vi "readEnc.vi"(0 "SPI Config In":T2) -> (1 "SPI Config Out":T2, 2 "Data Out":T1)   [LabVIEW 2019]
uses:
  SPI/SPI Config.ctl
panel:
  in  "Data Out Reference":T1
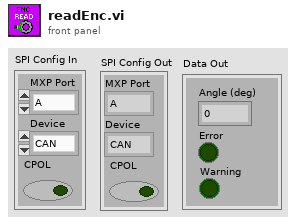
[diagram p1: front panel]
types:
  T1 = cluster{"Angle (deg)":fxp<+,32,16>, "Error":bool, "Warning":bool}
  T2 = typedef "SPI Config.ctl" = cluster{"MXP Port":enum16{"A", "B"}, "Device":enum16{"CAN", "ENC", "IMU1", "IMU2"}, "CPOL":bool}
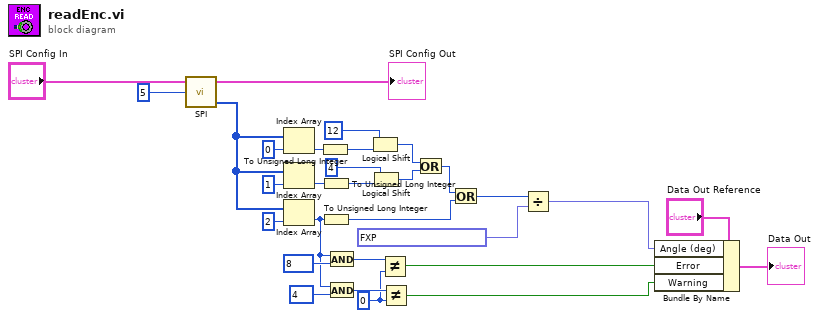
[diagram p0: block diagram]
diagram:
  w6 = u8 0 ("y")
  n1 = call "SPI.vi"("Frames to Write"=u8 5, "SPI Config In"="SPI Config In") -> ("Data Read"=w24:u8[], "SPI Config Out"=→"SPI Config Out":T2)  [unwired: 1 in, 1 out]
  n2 = Index Array(array=w24, index=0) -> (element=w23:u8)
  n3 = Index Array(array=w24, index=1) -> (element=w22:u8)
  n4 = Index Array(array=w24, index=2) -> (element=w10:u8)
  n5 = To Unsigned Long Integer(number=w23) -> (unsigned 32bit integer=w21:u32)
  n6 = To Unsigned Long Integer(number=w22) -> (unsigned 32bit integer=w20:u32)
  n7 = To Unsigned Long Integer(number=w10) -> (unsigned 32bit integer=w14:u32)
  n8 = And(x=w10, y=u8 8) -> (x .and. y?=w8:u8)
  n9 = And(x=w10, y=u8 4) -> (x .and. y?=w7:u8)
  n10 = Logical Shift(y=i16 12, x=w21) -> (x << y=w17:u32)
  n11 = Logical Shift(y=i16 4, x=w20) -> (x << y=w16:u32)
  n12 = Not Equal?(x=w8, y=w6) -> (x != y?=w4:bool)
  n13 = Not Equal?(x=w7, y=w6) -> (x != y?=w5:bool)
  n14 = Or(x=w17, y=w16) -> (x .or. y?=w15:u32)
  n15 = Or(x=w15, y=w14) -> (x .or. y?=w13:u32)
  n16 = Divide(x=w13, y=fxp<+,32,16> 2912.7083282470703) -> (x/y=w2:fxp<+,32,16>)
  n17 = Bundle By Name(cluster="Data Out Reference", "Angle (deg)"=w2, "Error"=w4, "Warning"=w5) -> (→"Data Out":T1)
